vi "Termék mentés.vi"(8 "error in":errorcluster, 11 "Termék cluster array":T1[](array[typedef])) -> (0 "error out":errorcluster, 3 "File name":string)   [LabVIEW 2014]
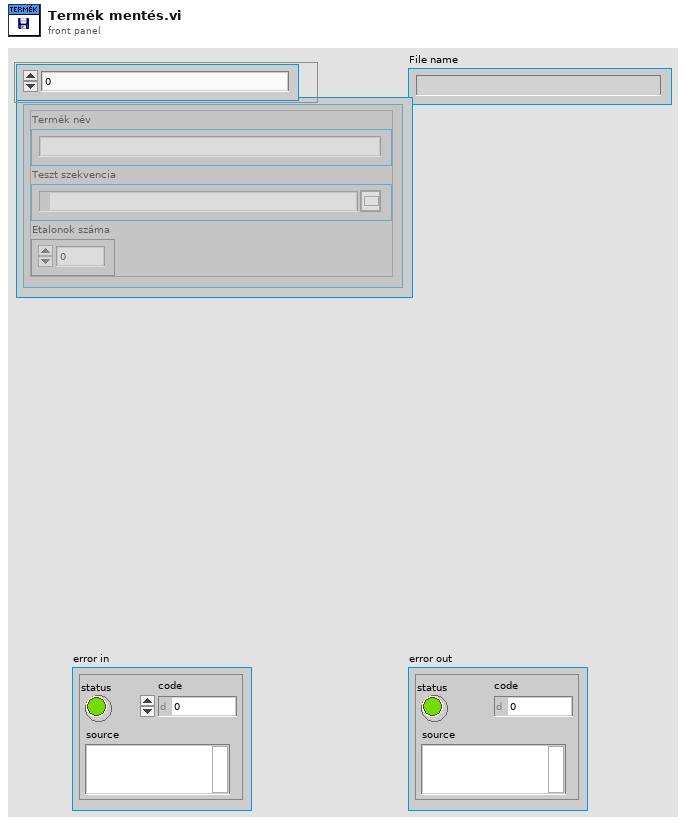
[diagram p1: front panel]
types:
  T1 = typedef "Termék cluster.ctl" = cluster{"Termék név":string, "Teszt szekvencia":path, "Etalonok száma":i8}
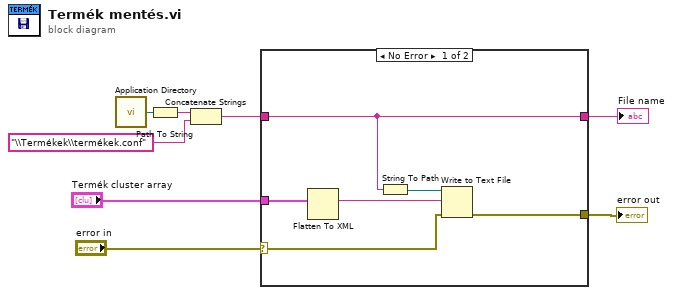
[diagram p0: block diagram]
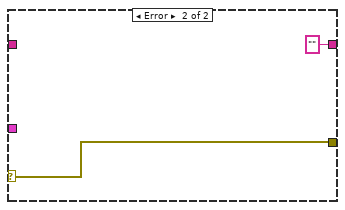
[diagram p2: hidden frame]
diagram:
  n1 = call <vilib>:"Application Directory.vi"() -> ("Application Directory"=w7:path)
  n2 = Path To String(path=w7) -> (string=w6:string)
  n3 = Concatenate Strings(w6, "\\Termékek\\termékek.conf" ("pattern (all files)")) -> (w2:string)
  n4 = case shown="No Error" "error in" {
    selector: "error in" -> [w9 w16]
    tunnel: [w13 w16] -> w8
    tunnel: "Termék cluster array" -> [w12 _]
    tunnel: w2 -> [w10 _]
    tunnel: [w10 ""] -> w1
    frame No Error {
      n5 = Flatten To XML(anything=w12) -> (xml string=w14:string)
      n6 = String To Path(string=w10) -> (path=w11:path)
      n7 = Write to Text File(file (use dialog)=w11, text=w14, error in=w9) -> (error out=w13:errorcluster)  [unwired: 1 in, 2 out]
    }
    frame Error {
    }
  }
  "error out" <- w8
  "File name" <- w1
